vi "Teszt szerkesztő2.vi"(11 "Teszt cluster in":T1) -> (3 "Teszt cluster out":T1)   [LabVIEW 2014]
uses:
  Teszt.ctl
  Command.ctl
panel:
  in  "Select":bool
  in  "Expand":bool
  in  "Collapse":bool
  in  "Tree":string(tree)
  in  "OK":bool
  in  "cancel":bool
  in  "Teszt cluster Temp":T1
  # "Parancs / Mérés Szerkesztõ"
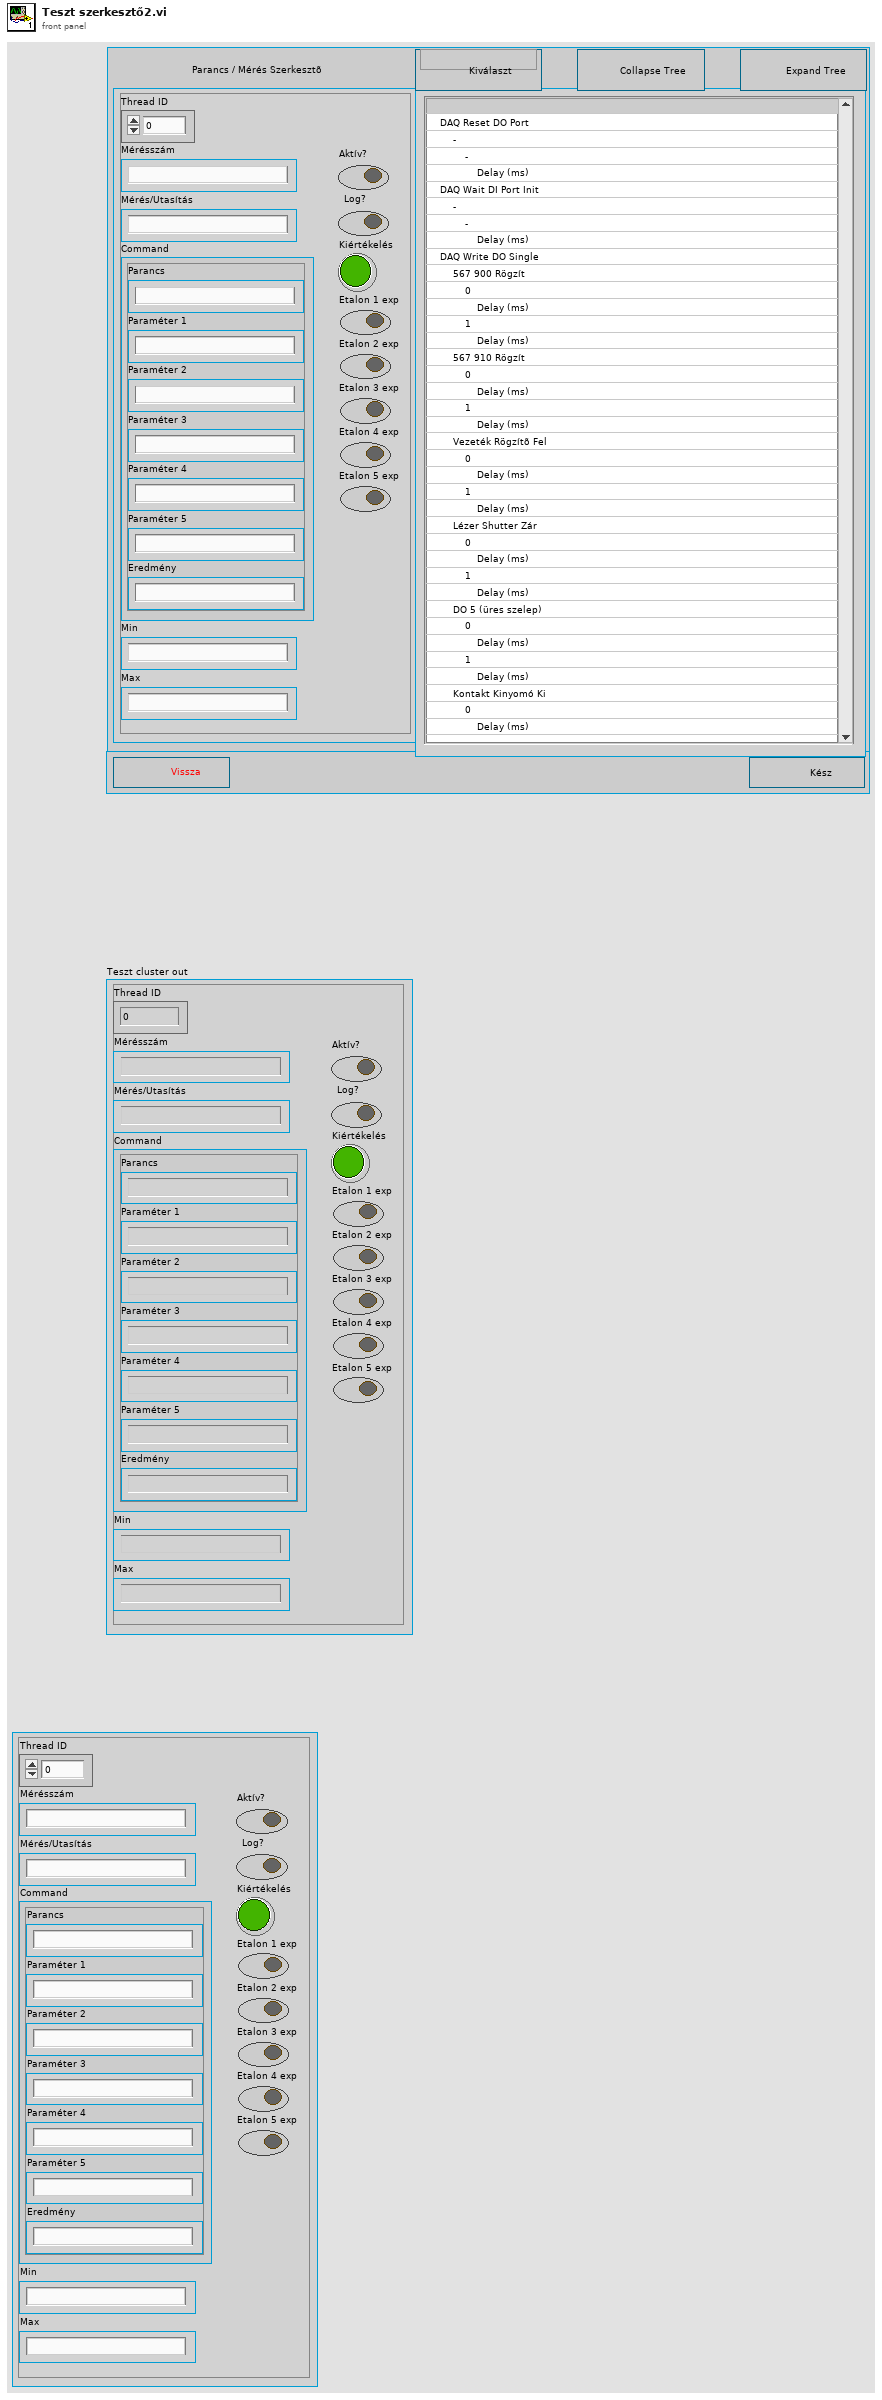
[diagram p1: front panel]
types:
  T1 = typedef "Teszt.ctl" = cluster{"Thread ID":dbl, "Mérésszám":string, "Mérés/Utasítás":string, "Command":T2, "Min":string, "Max":string, "Aktív?":bool, "Log?":bool, "Kiértékelés":bool, "Etalon 1 exp":bool, "Etalon 2 exp":bool, "Etalon 3 exp":bool, "Etalon 4 exp":bool, "Etalon 5 exp":bool}
  T2 = typedef "Command.ctl" = cluster{"Parancs":string, "Paraméter 1":string, "Paraméter 2":string, "Paraméter 3":string, "Paraméter 4":string, "Paraméter 5":string, "Eredmény":string}
  T3 = cluster{"[0]":string, "[1]":string, "[2]":string, "[3]":string, "[4]":string, "[5]":string, "[6]":string}
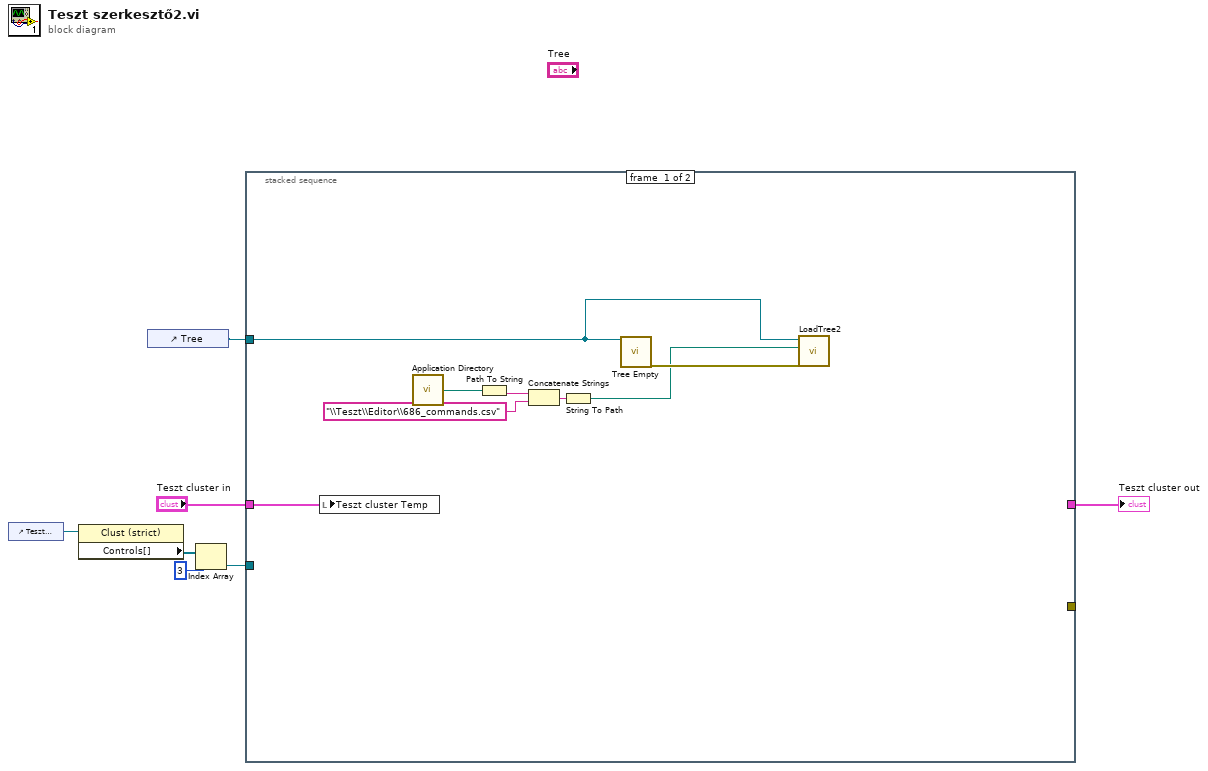
[diagram p0: block diagram]
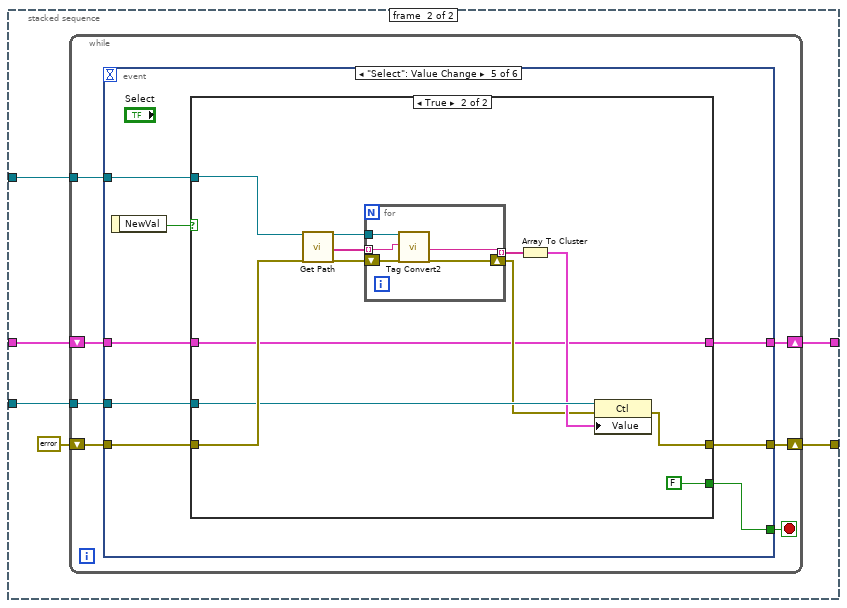
[diagram p2: hidden frame]
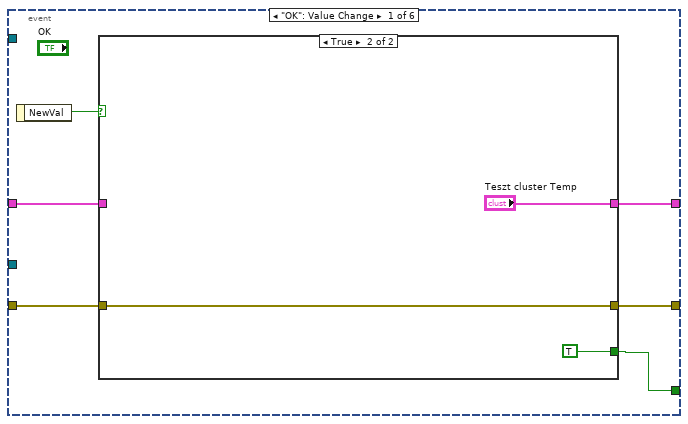
[diagram p3: hidden frame]
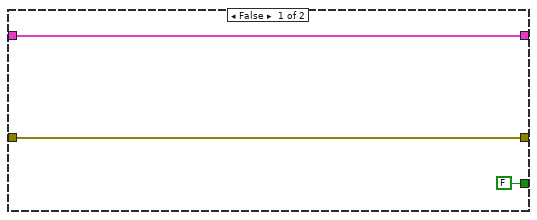
[diagram p4: hidden frame]
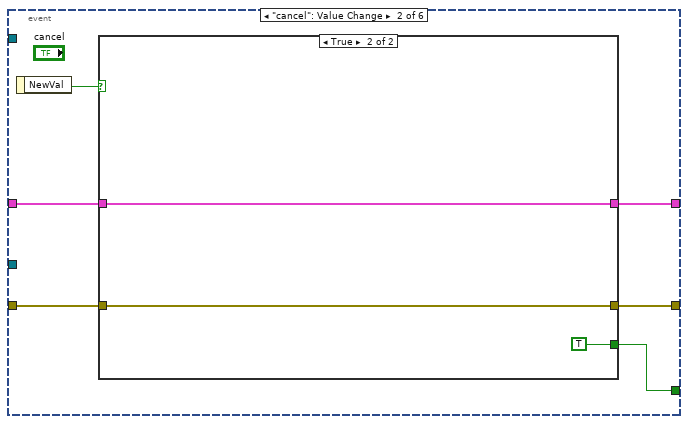
[diagram p5: hidden frame]
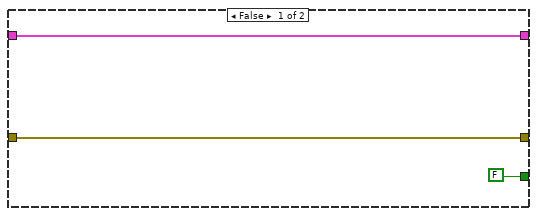
[diagram p6: hidden frame]
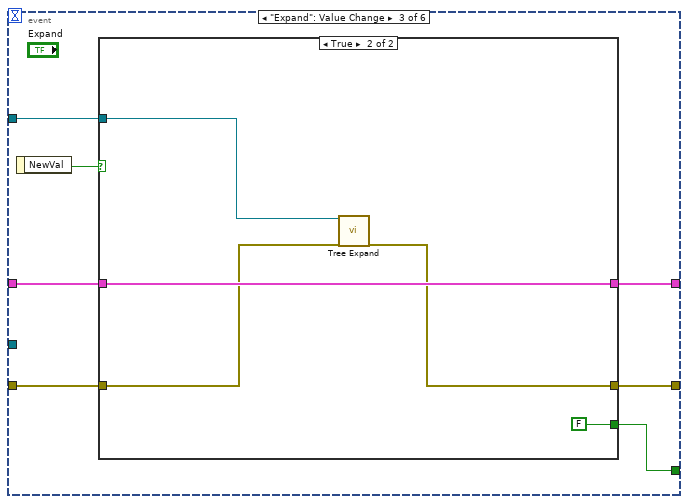
[diagram p7: hidden frame]
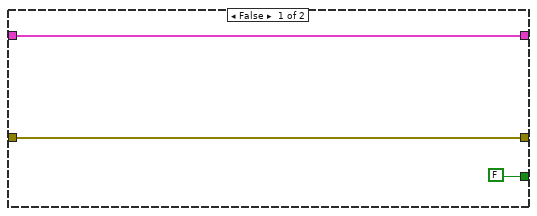
[diagram p8: hidden frame]
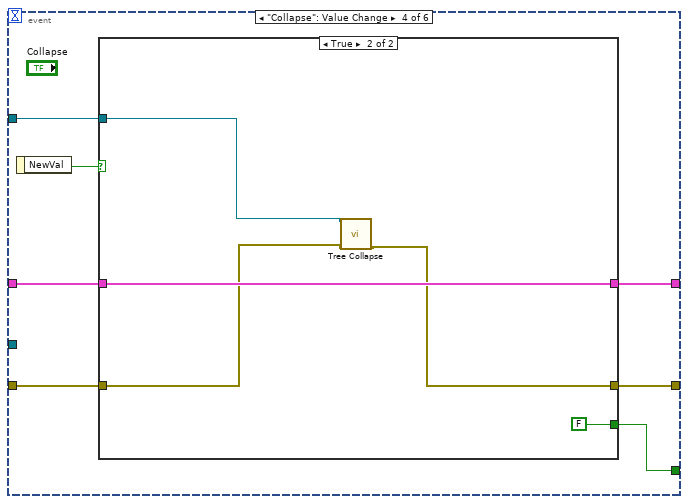
[diagram p9: hidden frame]
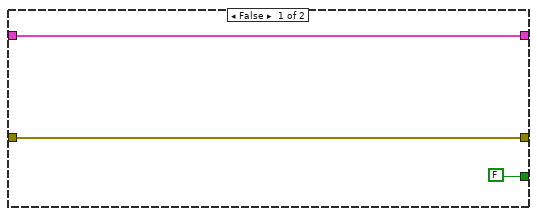
[diagram p10: hidden frame]
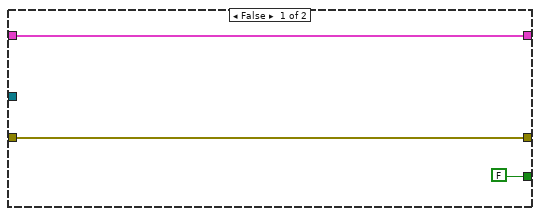
[diagram p11: hidden frame]
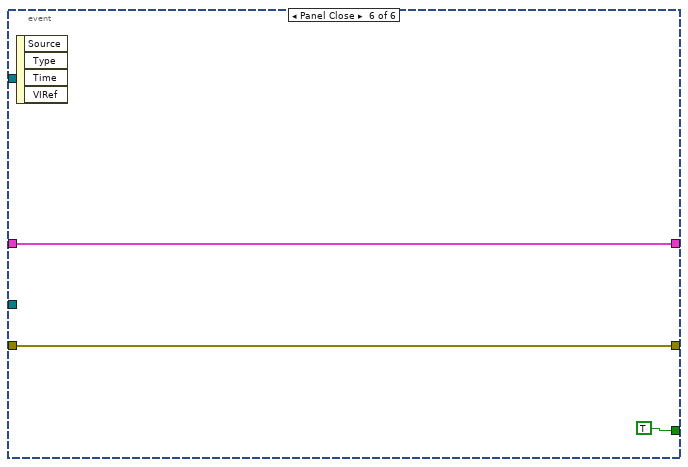
[diagram p12: hidden frame]
diagram:
  n1 = control-ref of="Teszt cluster Temp"() -> (w4:refnum<vi>)
  n2 = property class="Clust (strict)"(reference=w4) -> ("Controls[]"=w3:refnum<vi>[])  [unwired: 1 in, 2 out]
  n3 = control-ref of="Tree"() -> (w5:refnum<vi>)
  n4 = Index Array(array=w3, index=3) -> (element=w1:refnum<vi>)
  n5 = stacked-sequence {
    tunnel: "Teszt cluster in" -> [w15 w21]
    tunnel: [_ w20] -> w7
    tunnel: w5 -> [w10 w19]
    tunnel: w1 -> [_ w18]
    tunnel: [_ w17] -> _
    frame #0 {
      n6 = local write "Teszt cluster Temp"(w15) -> ()
      n7 = call <vilib>:"Application Directory.vi"() -> ("Application Directory"=w11:path)
      n8 = Path To String(path=w11) -> (string=w14:string)
      n9 = Concatenate Strings(w14, "\\Teszt\\Editor\\686_commands.csv" ("prompt (Choose or enter file path)")) -> (w13:string)
      n10 = String To Path(string=w13) -> (path=w8:path)
      n11 = call "Tree Empty.vi"("Tree Reference In"=w10) -> ("error out"=w9:errorcluster)  [unwired: 16 in, 2 out]
      n12 = call "LoadTree2.vi"("error in"=w9, "File Path Control"=w8, "TreeControl reference"=w10) -> ()  [unwired: 8 in, 1 out]
    }
    frame #1 {
      n13 = while {
        shift-right: [w27] -> w20
        shift-left: w21 -> [w28]
        tunnel: w19 -> [w25]
        shift-right: [w24] -> w17
        shift-left: errorcluster {"status"=FALSE, "code"=0, "source"=""} ("error out") -> [w23]
        tunnel: w18 -> [w22]
        stop <- w26 stop-if-true
        n14 = event shown="[4] \"Select\": Value Change" {
          selector: _ -> [_ _ _ _ _ _]
          dyn-events: _ -> [_ _ _ _ _ _]
          timeout: _ -> [_ _ _ _ _ _]
          tunnel: w28 -> [w33 w44 w57 w72 w88 w113]
          tunnel: [w32 w45 w58 w73 w89 w113] -> w27
          tunnel: [w31 w43 w56 w71 w87 TRUE] -> w26
          tunnel: w25 -> [_ _ w55 w70 w86 _]
          tunnel: [w29 w41 w54 w69 w85 w111] -> w24
          tunnel: w23 -> [w30 w42 w53 w68 w84 w111]
          tunnel: w22 -> [_ _ _ _ w83 _]
          event "OK": Value Change {
            n15 = event-data() -> ("NewVal"=w34:bool)  [unwired: 1 in]
            n16 = case shown="True" w34 {
              tunnel: w33 -> [w37 _]
              tunnel: [w37 "Teszt cluster Temp"] -> w32
              tunnel: [FALSE TRUE] -> w31
              tunnel: [w35 w38] -> w29
              tunnel: w30 -> [w35 w38]
              frame False {
              }
              frame True {
              }
            }
          }
          event "cancel": Value Change {
            n17 = event-data() -> ("NewVal"=w46:bool)  [unwired: 1 in]
            n18 = case shown="True" w46 {
              tunnel: [w49 w52] -> w45
              tunnel: w44 -> [w49 w52]
              tunnel: [FALSE TRUE] -> w43
              tunnel: [w47 w50] -> w41
              tunnel: w42 -> [w47 w50]
              frame False {
              }
              frame True {
              }
            }
          }
          event "Expand": Value Change {
            n19 = event-data() -> ("NewVal"=w59:bool)  [unwired: 1 in]
            n20 = case shown="True" w59 {
              tunnel: [w62 w67] -> w58
              tunnel: w57 -> [w62 w67]
              tunnel: [FALSE FALSE] -> w56
              tunnel: w55 -> [_ w65]
              tunnel: [w60 w64] -> w54
              tunnel: w53 -> [w60 w63]
              frame False {
              }
              frame True {
                n21 = call "Tree Expand.vi"("Tree Reference In"=w65, "error in (no error)"=w63) -> ("error out"=w64:errorcluster)  [unwired: 16 in, 1 out]
              }
            }
          }
          event "Collapse": Value Change {
            n22 = event-data() -> ("NewVal"=w74:bool)  [unwired: 1 in]
            n23 = case shown="True" w74 {
              tunnel: [w77 w82] -> w73
              tunnel: w72 -> [w77 w82]
              tunnel: [FALSE FALSE] -> w71
              tunnel: w70 -> [_ w79]
              tunnel: [w75 w78] -> w69
              tunnel: w68 -> [w75 w80]
              frame False {
              }
              frame True {
                n24 = call "Tree Collapse.vi"("Tree Reference In"=w79, "error in (no error)"=w80) -> ("error out"=w78:errorcluster)  [unwired: 16 in, 1 out]
              }
            }
          }
          event "Select": Value Change {
            n25 = event-data() -> ("NewVal"=w90:bool)  [unwired: 1 in]
            n26 = case shown="True" w90 {
              tunnel: [w93 w94] -> w89
              tunnel: w88 -> [w93 w94]
              tunnel: [FALSE FALSE] -> w87
              tunnel: w86 -> [_ w103]
              tunnel: [w91 w95] -> w85
              tunnel: w84 -> [w91 w104]
              tunnel: w83 -> [_ w98]
              frame False {
              }
              frame True {
                n27 = call "Get Path.vi"("Tree Reference In"=w103, "error in (no error)"=w104) -> ("Tree Reference Out"=w102:refnum<vi>, "Path"=w101:string[], "error out"=w100:errorcluster)  [unwired: 15 in]
                n28 = for {
                  tunnel: w102 -> [w110]
                  tunnel: w101 -> [w109] mode=indexing
                  shift-right: [w107] -> w96
                  shift-left: w100 -> [w108]
                  tunnel: [w106] -> w99 mode=indexing
                  n29 = call "Tag Convert2.vi"("Tree Reference In"=w110, "InputTag (Current)"=w109, "error in (no error)"=w108) -> ("Tag Text"=w106:string, "error out"=w107:errorcluster)  [unwired: 13 in, 2 out]
                }
                n30 = Array To Cluster(array=w99) -> (cluster=w97:T3)
                n31 = property class="Ctl"(reference=w98, error in=w96, "Value"=w97) -> (error out=w95:errorcluster)  [unwired: 1 out]
              }
            }
          }
          event Panel Close {
            n32 = event-data() -> ()  [unwired: 1 in, 4 out]
          }
        }
      }
    }
  }
  "Teszt cluster out" <- w7
